vi "ProbePlanAlign_Chuck.vi"(10 "New Sensor":bool, 11 "ProbeStationControl in":refnum<class "ProbeStationControl.lvclass">) -> (2 "Accept/Quit":bool, 3 "ProbeStationControl out":refnum<class "ProbeStationControl.lvclass">)   [LabVIEW 2013]
uses:
  InstrControl/ProbeStationControl/ProbeStationControl.lvclass
  ProbePlanParams.vi
panel:
  in  "Old reference":bool
  in  "Already aligned":bool
  in  "align":bool
  out "Y1 2":i32
  out "X1 2":i32
  in  "Read probeplan reference":bool
  out "Y1280":i32
  out "X1280":i32
  in  "Readtop fiducial":bool
  out "Y1":i32
  out "X1":i32
  in  "Quit":bool
  in  "Accept":bool
  in  "Read bottom fiducial":bool
  # "Map Sensor to ProbePlan"
  # "X"
  # "Y"
  # "First Step:Align the sensor"
  # "as reference for bottom fiducial"
  # "as reference for top fiducial"
  # "Second step: locate the probeplan reference point on the sensor"
  # "as reference for ProbePlan"
  # "X:"
  # "Y:"
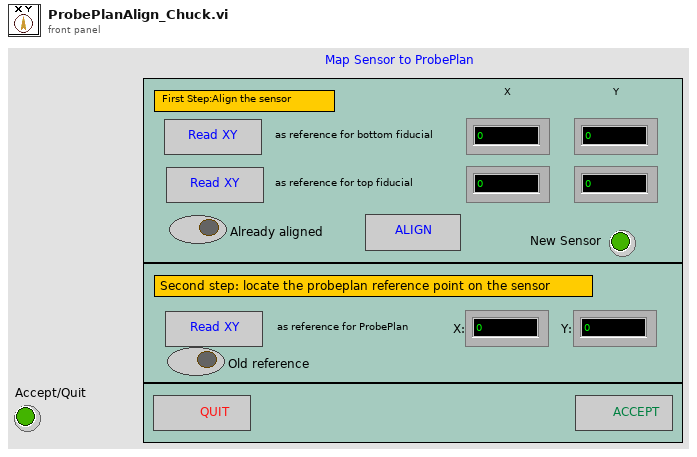
[diagram p1: front panel]
types:
  T1 = cluster{"Strip Number OUT":i32, "X0":i32, "Y0":i32, "X1":i32, "Y1":i32, "Xref":dbl, "Yref":dbl, "ProbePlan type":u32, "Inner pads offset":ext, "Outer pads offset":ext, "l_inner":ext, "l_outer":ext, "strip numbering":u16, "Device Orientation":ext, "Stagger offset":i32, "Yoffset":dbl, "Strip pitch":dbl, "Fiducail separation":dbl, "Radius":ext, "Relative strip angles":dbl, "Probeplan description":string, "ProbePlan array":cluster{"Region":string, "ProbePoints":cluster{"X":dbl, "Y":dbl, "Label":string, "CardViable?":bool}[]}[], "Test ProbePoints":cluster{"Regions Enabled":bool[], "From index":u32[], "To index":u32[]}}
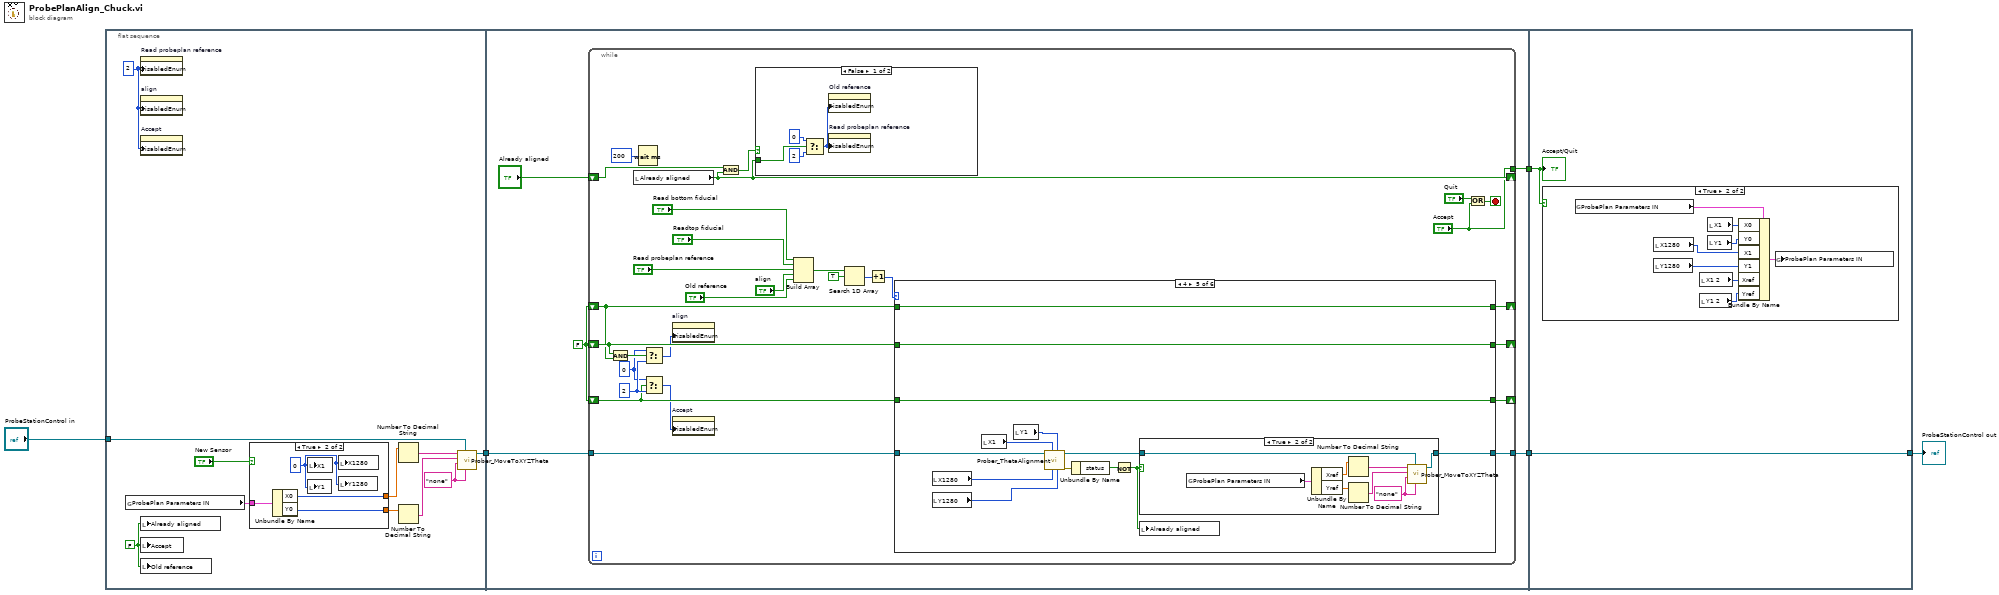
[diagram p0: block diagram]
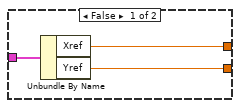
[diagram p2: hidden frame]
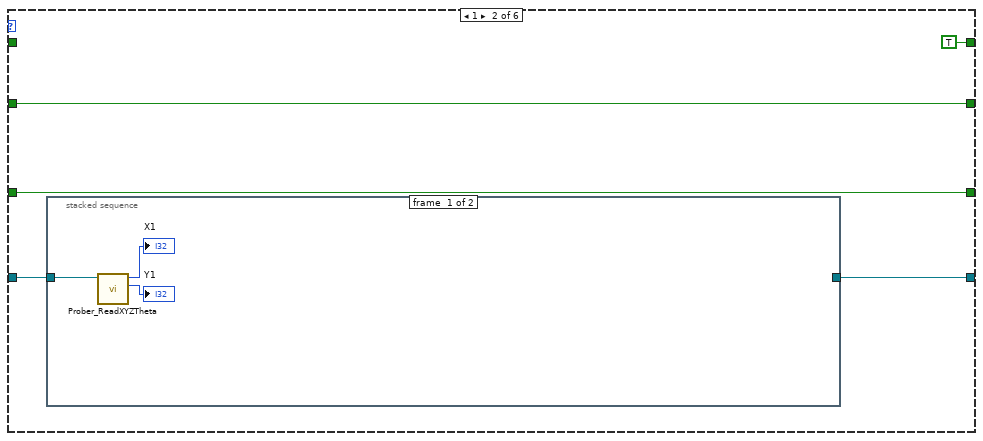
[diagram p4: hidden frame]
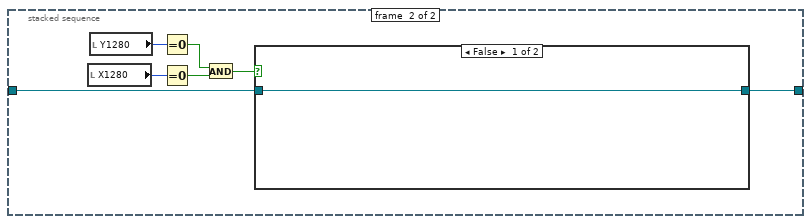
[diagram p5: hidden frame]
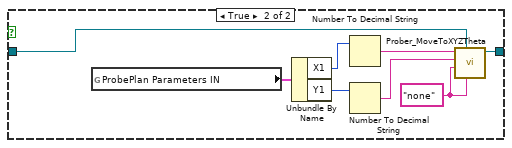
[diagram p6: hidden frame]
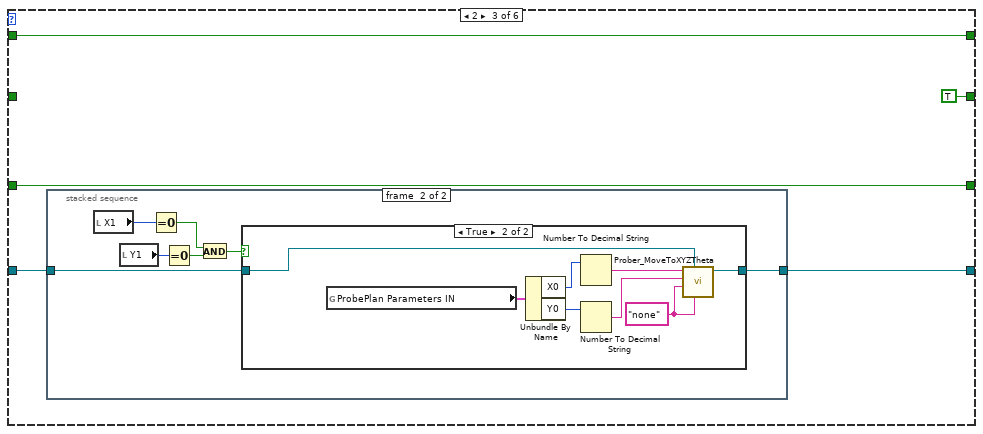
[diagram p7: hidden frame]
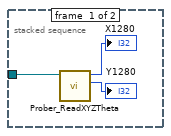
[diagram p8: hidden frame]
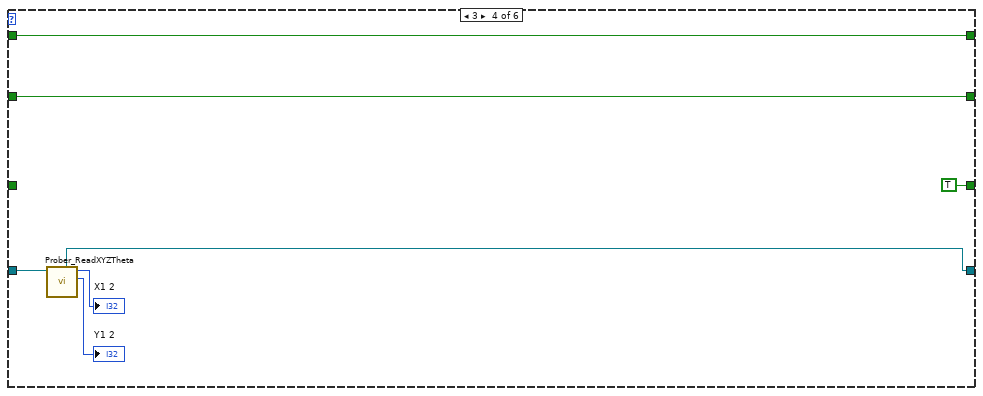
[diagram p10: hidden frame]
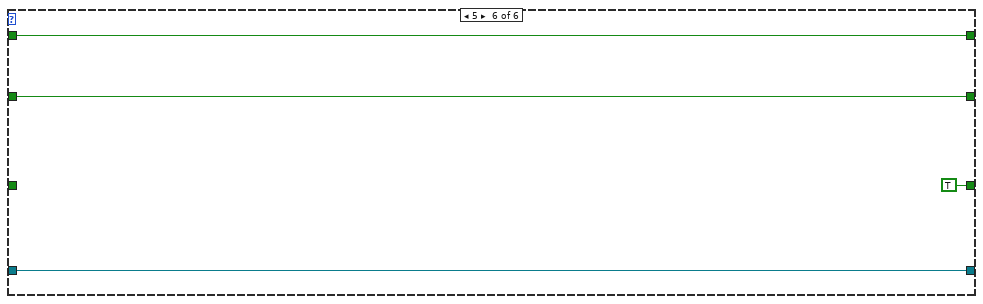
[diagram p12: hidden frame]
diagram:
  n1 = flat-sequence {
    tunnel: "ProbeStationControl in" -> [w7]
    tunnel: [w6] -> w3
    tunnel: [w27] -> w5
    tunnel: w3 -> [w25]
    tunnel: [w24] -> w2
    tunnel: w5 -> [w148]
    tunnel: w2 -> [w147]
    tunnel: [w147] -> w1
    frame #0 {
      w14 = "none"
      w16 = 2
      w15 = FALSE
      n2 = global read "ProbePlanParams.vi" "ProbePlan Parameters IN"() -> (w10:T1)
      n3 = property on="Read probeplan reference" class="Bool"("DisabledEnum"=w16) -> ()  [unwired: 2 in, 2 out]
      n4 = property on="align" class="Bool"("DisabledEnum"=w16) -> ()  [unwired: 2 in, 2 out]
      n5 = property on="Accept" class="Bool (strict)"("DisabledEnum"=w16) -> ()  [unwired: 2 in, 2 out]
      n6 = local write "Already aligned"(w15) -> ()
      n7 = local write "Accept"(w15) -> ()
      n8 = local write "Old reference"(w15) -> ()
      n9 = case shown="True" "New Sensor" {
        tunnel: w10 -> [w19 w23]
        tunnel: [w18 w22] -> w9
        tunnel: [w17 w21] -> w8
        frame False {
          n10 = Unbundle By Name(w19) -> ("Xref"=w18:dbl, "Yref"=w17:dbl)
        }
        frame True {
          w20 = 0
          n11 = Unbundle By Name(w23) -> ("X0"=w22:i32, "Y0"=w21:i32)
          n12 = local write "X1"(w20) -> ()
          n13 = local write "Y1"(w20) -> ()
          n14 = local write "X1280"(w20) -> ()
          n15 = local write "Y1280"(w20) -> ()
        }
      }
      n16 = Number To Decimal String(number=w9) -> (decimal integer string=w13:string)  [unwired: 1 in]
      n17 = Number To Decimal String(number=w8) -> (decimal integer string=w12:string)  [unwired: 1 in]
      n18 = call-dynamic "Prober_MoveToXYZTheta.vi"("Theta location [mdeg]"=w14, "ProbeStationControl in"=w7, "Z location [µm]"=w14, "Y location [µm]"=w12, "X location [µm]"=w13) -> ("ProbeStationControl out"=w6:refnum<class "ProbeStationControl.lvclass">)  [unwired: 4 in, 2 out]
    }
    frame #1 {
      w26 = FALSE
      n19 = while {
        shift-right: [w56] -> _
        shift-left: "Already aligned" -> [w42]
        tunnel: ["Accept"] -> w27
        shift-right: [w41] -> _
        shift-left: w26 -> [w44]
        shift-right: [w39] -> _
        shift-left: w26 -> [w30]
        shift-right: [w40] -> _
        shift-left: w26 -> [w43]
        tunnel: w25 -> [w36]
        tunnel: [w35] -> w24
        stop <- w54 stop-if-true
        w32 = 2
        w31 = 0
        n20 = And(x=w44, y=w43) -> (x .and. y?=w34:bool)
        n21 = local read "Already aligned"() -> (w56:bool)
        n22 = Wait (ms)(milliseconds to wait=u32 200) -> ()  [unwired: 1 out]
        n23 = Select(t=w31, s=w34, f=w32) -> (s? t:f=w33:i32)
        n24 = Select(t=w31, s=w30, f=w32) -> (s? t:f=w29:i32)
        n25 = property on="align" class="Bool"("DisabledEnum"=w33) -> ()  [unwired: 2 in, 2 out]
        n26 = property on="Accept" class="Bool (strict)"("DisabledEnum"=w29) -> ()  [unwired: 2 in, 2 out]
        n27 = And(x=w42, y=w56) -> (x .and. y?=w57:bool)
        n28 = case shown="False" w57 {
          tunnel: w56 -> [w144 _]
          frame False {
            n29 = Select(t=0, s=w144, f=2) -> (s? t:f=w143:i32)
            n30 = property on="Old reference" class="Bool (strict)"("DisabledEnum"=w143) -> ()  [unwired: 2 in, 2 out]
            n31 = property on="Read probeplan reference" class="Bool"("DisabledEnum"=w143) -> ()  [unwired: 2 in, 2 out]
          }
          frame True {
          }
        }
        n32 = Build Array("Read bottom fiducial", "Readtop fiducial", "Read probeplan reference", "align", "Old reference") -> (w47:bool[])
        n33 = Search 1D Array(1D array=w47, element=TRUE) -> (index of element=w46:i32)  [unwired: 1 in]
        n34 = Increment(x=w46) -> (x+1=w45:i32)
        n35 = case shown="4" w45 {
          tunnel: w44 -> [w60 w64 _ w113 w124 w141]
          tunnel: w43 -> [w59 _ w90 w112 w125 w140]
          tunnel: [w60 w64 TRUE w113 w124 w141] -> w41
          tunnel: [w59 TRUE w90 w112 w125 w140] -> w40
          tunnel: w30 -> [w61 w66 w88 _ w123 _]
          tunnel: [w61 w66 w88 TRUE w123 TRUE] -> w39
          tunnel: w36 -> [w58 w63 w87 w111 w122 w139]
          tunnel: [w58 w62 w86 w110 w120 w139] -> w35
          frame 0, Default {
          }
          frame 1 {
            n36 = stacked-sequence {
              tunnel: w63 -> [w67 w70]
              tunnel: [_ w71] -> w62
              frame #0 {
                n37 = call-dynamic "Prober_ReadXYZTheta.vi"("ProbeStationControl in"=w67) -> ("Y location [µm]"=→"Y1":i32, "X location [µm]"=→"X1":i32)  [unwired: 5 in, 4 out]
              }
              frame #1 {
                n38 = local read "X1280"() -> (w76:i32)
                n39 = local read "Y1280"() -> (w75:i32)
                n40 = Equal To 0?(x=w75) -> (x = 0?=w74:bool)
                n41 = Equal To 0?(x=w76) -> (x = 0?=w73:bool)
                n42 = And(x=w74, y=w73) -> (x .and. y?=w72:bool)
                n43 = case shown="False" w72 {
                  tunnel: w70 -> [w77 w79]
                  tunnel: [w77 w78] -> w71
                  frame False {
                  }
                  frame True {
                    w80 = "none"
                    n44 = global read "ProbePlanParams.vi" "ProbePlan Parameters IN"() -> (w83:T1)
                    n45 = Unbundle By Name(w83) -> ("X1"=w84:i32, "Y1"=w85:i32)
                    n46 = Number To Decimal String(number=w84) -> (decimal integer string=w81:string)  [unwired: 1 in]
                    n47 = Number To Decimal String(number=w85) -> (decimal integer string=w82:string)  [unwired: 1 in]
                    n48 = call-dynamic "Prober_MoveToXYZTheta.vi"("Theta location [mdeg]"=w80, "ProbeStationControl in"=w79, "Z location [µm]"=w80, "Y location [µm]"=w82, "X location [µm]"=w81) -> ("ProbeStationControl out"=w78:refnum<class "ProbeStationControl.lvclass">)  [unwired: 4 in, 2 out]
                  }
                }
              }
            }
          }
          frame 2 {
            n49 = stacked-sequence {
              tunnel: w87 -> [w91 w94]
              tunnel: [_ w95] -> w86
              frame #0 {
                n50 = call-dynamic "Prober_ReadXYZTheta.vi"("ProbeStationControl in"=w91) -> ("Y location [µm]"=→"Y1280":i32, "X location [µm]"=→"X1280":i32)  [unwired: 5 in, 4 out]
              }
              frame #1 {
                n51 = local read "X1"() -> (w100:i32)
                n52 = local read "Y1"() -> (w99:i32)
                n53 = Equal To 0?(x=w100) -> (x = 0?=w97:bool)
                n54 = Equal To 0?(x=w99) -> (x = 0?=w98:bool)
                n55 = And(x=w97, y=w98) -> (x .and. y?=w96:bool)
                n56 = case shown="True" w96 {
                  tunnel: [w101 w103] -> w95
                  tunnel: w94 -> [w101 w102]
                  frame False {
                  }
                  frame True {
                    w104 = "none"
                    n57 = global read "ProbePlanParams.vi" "ProbePlan Parameters IN"() -> (w107:T1)
                    n58 = Unbundle By Name(w107) -> ("X0"=w108:i32, "Y0"=w109:i32)
                    n59 = Number To Decimal String(number=w108) -> (decimal integer string=w105:string)  [unwired: 1 in]
                    n60 = Number To Decimal String(number=w109) -> (decimal integer string=w106:string)  [unwired: 1 in]
                    n61 = call-dynamic "Prober_MoveToXYZTheta.vi"("Theta location [mdeg]"=w104, "ProbeStationControl in"=w102, "Z location [µm]"=w104, "Y location [µm]"=w106, "X location [µm]"=w105) -> ("ProbeStationControl out"=w103:refnum<class "ProbeStationControl.lvclass">)  [unwired: 4 in, 2 out]
                  }
                }
              }
            }
          }
          frame 3 {
            n62 = call-dynamic "Prober_ReadXYZTheta.vi"("ProbeStationControl in"=w111) -> ("Y location [µm]"=→"Y1 2":i32, "X location [µm]"=→"X1 2":i32, "ProbeStationControl out"=w110:refnum<class "ProbeStationControl.lvclass">)  [unwired: 5 in, 3 out]
          }
          frame 4 {
            n63 = local read "X1280"() -> (w129:i32)
            n64 = local read "Y1280"() -> (w126:i32)
            n65 = local read "X1"() -> (w128:i32)
            n66 = local read "Y1"() -> (w127:i32)
            n67 = call-dynamic "Prober_ThetaAlignment.vi"("y2"=w126, "y1"=w127, "x2"=w129, "x1"=w128, "ProbeStationControl in"=w122) -> ("error out"=w119:errorcluster, "ProbeStationControl out"=w121:refnum<class "ProbeStationControl.lvclass">)  [unwired: 3 in, 2 out]
            n68 = Unbundle By Name(w119) -> ("status"=w118:bool)
            n69 = Not(x=w118) -> (.not. x?=w117:bool)
            n70 = case shown="True" w117 {
              tunnel: w121 -> [w130 w132]
              tunnel: [w130 w131] -> w120
              frame False {
              }
              frame True {
                w133 = "none"
                n71 = global read "ProbePlanParams.vi" "ProbePlan Parameters IN"() -> (w136:T1)
                n72 = Unbundle By Name(w136) -> ("Xref"=w137:dbl, "Yref"=w138:dbl)
                n73 = Number To Decimal String(number=w137) -> (decimal integer string=w134:string)  [unwired: 1 in]
                n74 = Number To Decimal String(number=w138) -> (decimal integer string=w135:string)  [unwired: 1 in]
                n75 = call-dynamic "Prober_MoveToXYZTheta.vi"("Theta location [mdeg]"=w133, "ProbeStationControl in"=w132, "Z location [µm]"=w133, "Y location [µm]"=w135, "X location [µm]"=w134) -> ("ProbeStationControl out"=w131:refnum<class "ProbeStationControl.lvclass">)  [unwired: 4 in, 2 out]
              }
            }
            n76 = local write "Already aligned"(w117) -> ()
          }
          frame 5 {
          }
        }
        n77 = Or(x="Quit", y="Accept") -> (x .or. y?=w54:bool)
      }
    }
    frame #2 {
      n78 = case shown="True" w148 {
        frame False {
        }
        frame True {
          n79 = global read "ProbePlanParams.vi" "ProbePlan Parameters IN"() -> (w153:T1)
          n80 = local read "X1280"() -> (w150:i32)
          n81 = local read "Y1280"() -> (w149:i32)
          n82 = local read "X1 2"() -> (w155:i32)
          n83 = local read "Y1 2"() -> (w154:i32)
          n84 = local read "X1"() -> (w152:i32)
          n85 = local read "Y1"() -> (w151:i32)
          n86 = Bundle By Name(cluster=w153, "X0"=w152, "Y0"=w151, "X1"=w150, "Y1"=w149, "Xref"=w155, "Yref"=w154) -> (w156:T1)
          n87 = global write "ProbePlanParams.vi" "ProbePlan Parameters IN"(w156) -> ()
        }
      }
      "Accept/Quit" <- w148
    }
  }
  "ProbeStationControl out" <- w1
